vi "Error_Logger.vi"(11 "Error_In":errorcluster) -> (4 "Error_Table":string[][](table) caption="Error Table", 15 "Error_Out":errorcluster)   [LabVIEW 2023]
doc: "This VI Shows the Error data of current and temperature."
uses:
  Controls/Error_Data.ctl
  Controls/Main_Status.ctl
  Controls/Queue_Operation.ctl
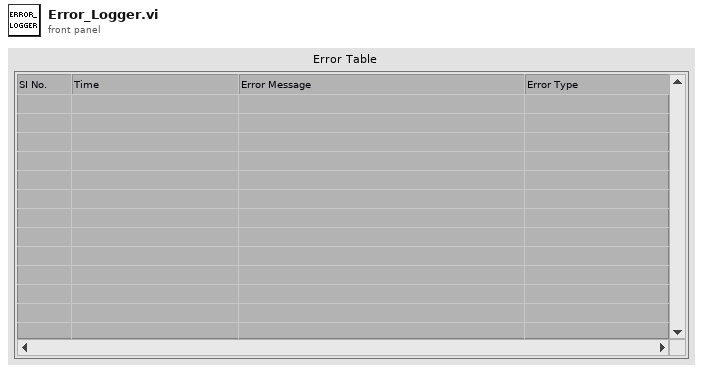
[diagram p1: front panel]
types:
  T1 = typedef "Main_Status.ctl" = cluster{"Stop?":bool, "Start/Stop_Acquisition ":bool, "Wait_Time":i32}
  T2 = enum32{"Invalid", "Standard", "Closed", "Hidden", "Minimized", "Maximized"}
  T3 = typedef "Error_Data.ctl" = cluster{"Error_Table_Data":string[][], "SI_No":i32}
  T4 = typedef "Queue_Operation.ctl" = enum16{"Obtain_Queue", "Enqueue", "Lossy_Enqueue", "Preview", "Queue_Status", "Release_Queue", "Dequeue", "Flush"}
  T5 = typedef "Logger_Data.ctl" = cluster{"Generated_Data":T6, "Current_Limit":T7, "Temperature_Limit":T8}
  T6 = typedef "Generated_data.ctl" = cluster{"Current_Data":dbl, "Temp_Data":dbl}
  T7 = typedef "Current_Limit.ctl" = cluster{"Current_High_Limit":dbl, "Current_Low_Limit":dbl}
  T8 = typedef "Temperature_Limit.ctl" = cluster{"Temperature_High_Limit":dbl, "Temperature_Low_Limit":dbl}
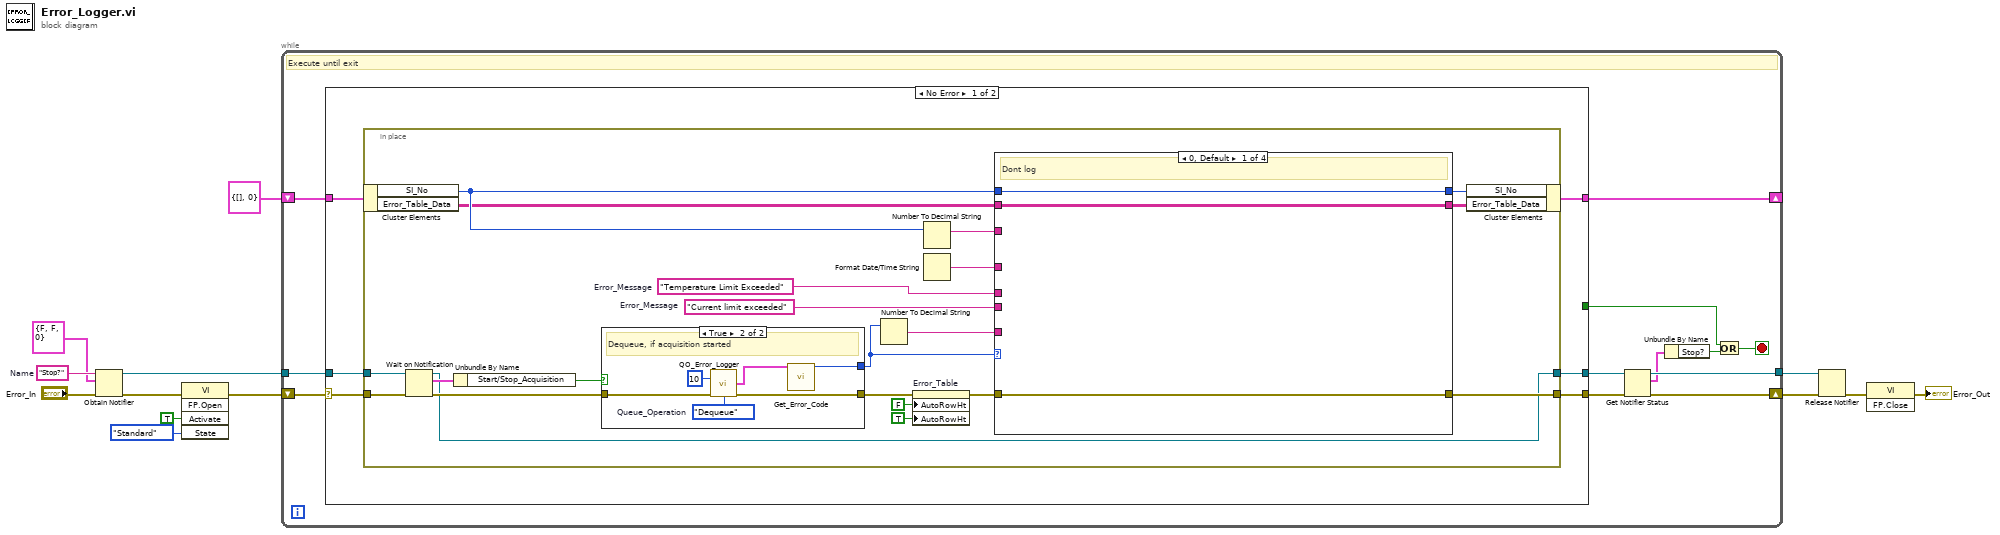
[diagram p0: block diagram]
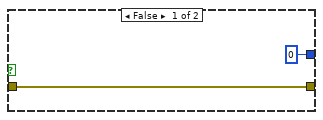
[diagram p2: hidden frame]
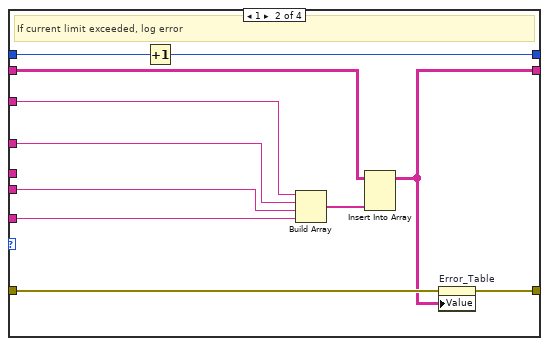
[diagram p3: hidden frame]
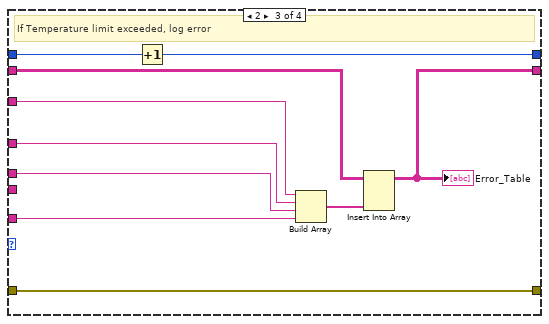
[diagram p4: hidden frame]
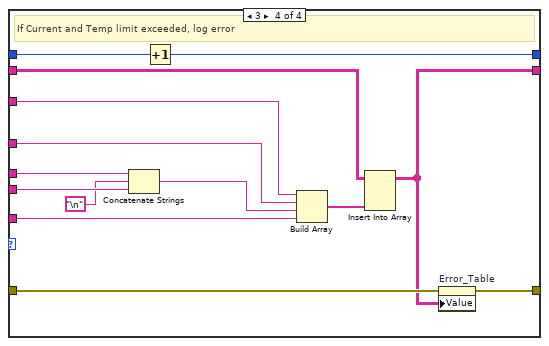
[diagram p5: hidden frame]
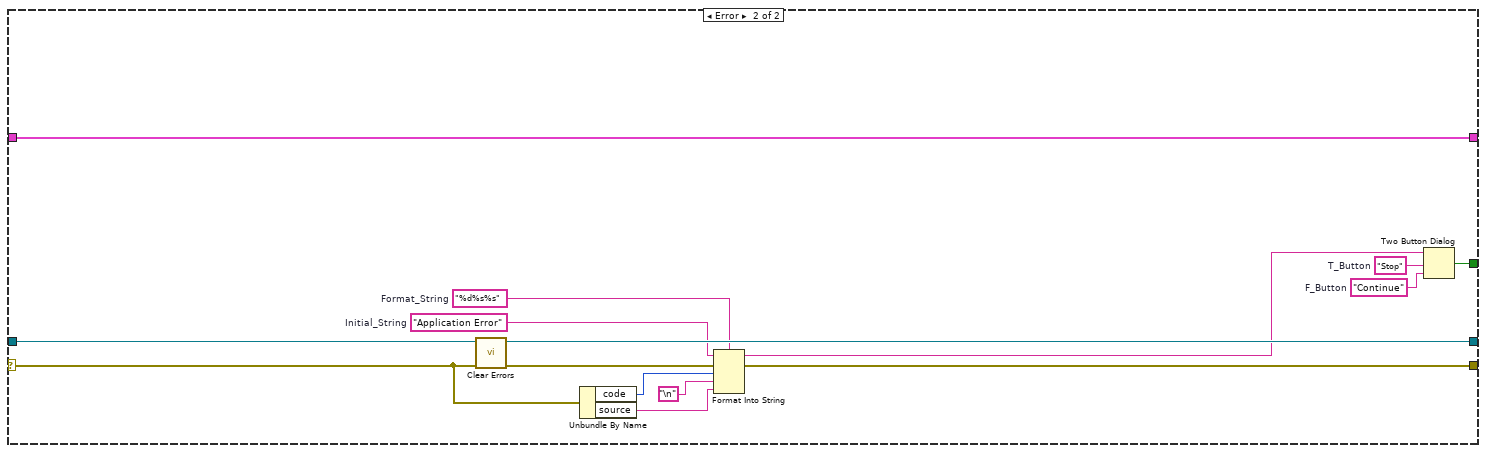
[diagram p6: hidden frame]
diagram:
  w9 = "Stop?"  # Name
  n1 = Obtain Notifier(name (unnamed)=w9, notification data type=T1 {"Stop?"=FALSE, "Start/Stop_Acquisition "=FALSE, "Wait_Time"=0} ("Cluster"), error in (no error)="Error_In") -> (notifier out=w8:refnum<notifier>, error out=w10:errorcluster)  [unwired: 1 in, 1 out]
  n2 = invoke class="VI" method="FP.Open"(error in=w10, "Activate"=TRUE ("Activate?"), "State"=T2."Standard") -> (error out=w4:errorcluster)  [unwired: 2 in, 4 out]
  n3 = while {
    shift-right: [w23] -> _
    shift-left: T3 {"Error_Table_Data"=[], "SI_No"=0} -> [w24]
    shift-right: [w21] -> w11
    shift-left: w4 -> [w25]
    tunnel: w8 -> [w19]
    tunnel: [w20] -> w7
    stop <- w15 stop-if-true
    # "Execute until exit"
    n4 = case shown="No Error" w25 {
      selector: w25 -> [w31 w102]
      tunnel: [w30 w103] -> w22
      tunnel: w24 -> [w29 w112]
      tunnel: [w28 w112] -> w23
      tunnel: w19 -> [w27 w111]
      tunnel: [w26 w111] -> w18
      tunnel: [_ w99] -> w14
      frame No Error {
        n5 = in-place {
          in-place-border: w31 -> [w52]
          in-place-border: [w49] -> w30
          in-place-border: w27 -> [w37]
          in-place-border: [w34] -> w26
          w41 = "Current limit exceeded"  # Error_Message
          w42 = "Temperature Limit Exceeded"  # Error_Message
          n6 = in-place-cluster #1(w29) -> ("SI_No"=w47:i32, "Error_Table_Data"=w46:string[][])
          n7 = Wait on Notification(notifier=w37, error in (no error)=w52) -> (notifier out=w34:refnum<notifier>, notification=w35:T1, error out=w38:errorcluster)  [unwired: 2 in, 1 out]
          n8 = Unbundle By Name(w35) -> ("Start/Stop_Acquisition"=w33:bool)
          n9 = case shown="True" w33 {
            tunnel: [w54 w59] -> w48
            tunnel: w38 -> [w54 w58]
            tunnel: [u32 0 ("Error_Code") w57] -> w32
            frame False {
            }
            frame True {
              w60 = Queue_Operation."Dequeue"  # Queue_Operation
              # "Dequeue, if acquisition started"
              n10 = call "QO_Error_Logger.vi"("Time_Out_In_ms (-1)"=10, "Error_In"=w58, "Queue_Operation"=w60) -> ("Data_Out"=w56:T5, "Error_Out"=w59:errorcluster)  [unwired: 8 in, 3 out]
              n11 = call "Get_Error_Code.vi"("Logger_Data"=w56) -> ("Error_Code"=w57:u32)  [unwired: 14 in]
            }
          }
          n12 = Number To Decimal String(number=w32) -> (decimal integer string=w43:string)  [unwired: 1 in]
          n13 = property on="Error_Table" class="Tbl (strict)"(error in=w48, "AutoRowHt"=FALSE ("Autosizing Row Height"), "AutoRowHt"=TRUE ("Autosizing Row Height")) -> (error out=w36:errorcluster)  [unwired: 1 in, 1 out]
          n14 = Number To Decimal String(number=w47) -> (decimal integer string=w51:string)  [unwired: 1 in]
          n15 = Format Date/Time String() -> (date/time string=w50:string)  [unwired: 3 in]
          n16 = case shown="0, Default" w32 {
            tunnel: w46 -> [w63 w74 w84 w98]
            tunnel: [w63 w64 w83 w90] -> w44
            tunnel: [w62 w73 w82 w97] -> w45
            tunnel: w47 -> [w62 w72 w81 w96]
            tunnel: w51 -> [_ w71 w80 w95]
            tunnel: w50 -> [_ w69 w78 w93]
            tunnel: [w61 w67 w77 w91] -> w49
            tunnel: w36 -> [w61 w68 w77 w92]
            tunnel: w43 -> [_ w66 w76 w89]
            tunnel: w42 -> [_ _ w75 w88]
            tunnel: w41 -> [_ w65 _ w86]
            frame 0, Default {
              # "Dont log"
            }
            frame 1 {
              # "If current limit exceeded, log error"
              n17 = Increment(x=w72) -> (x+1=w73:i32)
              n18 = Build Array(w71, w69, w65, w66) -> (w70:string[])
              n19 = Insert Into Array(array=w74, new element=w70) -> (w64:string[][])  [unwired: 2 in]
              n20 = property on="Error_Table" class="Tbl (strict)"(error in=w68, "Value"=w64) -> (error out=w67:errorcluster)  [unwired: 1 in, 1 out]
            }
            frame 2 {
              # "If Temperature limit exceeded, log error"
              n21 = Increment(x=w81) -> (x+1=w82:i32)
              n22 = Build Array(w80, w78, w75, w76) -> (w79:string[])
              n23 = Insert Into Array(array=w84, new element=w79) -> (w83:string[][])  [unwired: 2 in]
              "Error_Table" <- w83
            }
            frame 3 {
              # "If Current and Temp limit exceeded, log error"
              n24 = Concatenate Strings(w88, "\n", w86) -> (w87:string)
              n25 = Increment(x=w96) -> (x+1=w97:i32)
              n26 = Build Array(w95, w93, w87, w89) -> (w94:string[])
              n27 = Insert Into Array(array=w98, new element=w94) -> (w90:string[][])  [unwired: 2 in]
              n28 = property on="Error_Table" class="Tbl (strict)"(error in=w92, "Value"=w90) -> (error out=w91:errorcluster)  [unwired: 1 in, 1 out]
            }
          }
          n29 = in-place-cluster #1("SI_No"=w45, "Error_Table_Data"=w44) -> (w28:T3)
        }
      }
      frame Error {
        w106 = "%d%s%s"  # Format_String
        w107 = "Application Error"  # Initial_String
        w108 = "Stop"  # T_Button
        w109 = "Continue"  # F_Button
        n30 = call <vilib>:"Clear Errors.vi"("error in (no error)"=w102) -> ("error out"=w104:errorcluster)  [unwired: 5 in, 1 out]
        n31 = Unbundle By Name(w102) -> ("code"=w101:i32, "source"=w100:string)
        n32 = Format Into String(format string=w106, initial string=w107, error in=w104, w101, "\n", w100) -> (resulting string=w110:string, error out=w103:errorcluster)
        n33 = Two Button Dialog(message=w110, 1:w109, 2:w108) -> (T button?=w99:bool)
      }
    }
    n34 = Get Notifier Status(notifier=w18, error in (no error)=w22) -> (notifier out=w20:refnum<notifier>, current notification=w17:T1, error out=w21:errorcluster)  [unwired: 2 out]
    n35 = Unbundle By Name(w17) -> ("Stop?"=w16:bool)
    n36 = Or(x=w14, y=w16) -> (x .or. y?=w15:bool)
  }
  n37 = Release Notifier(notifier=w7, error in (no error)=w11) -> (error out=w6:errorcluster)  [unwired: 1 in, 2 out]
  n38 = invoke class="VI" method="FP.Close"(error in=w6) -> (error out=→"Error_Out":errorcluster)  [unwired: 2 in, 2 out]
